vi "SetKparAxisMax.vi"(8 "error in (no error)":errorcluster, 9 "newMax":dbl, 10 "kPar":i32, 11 "dvotAFTKinetics in":refnum<class "dvotAFTKinetics.lvclass">) -> (0 "error out":errorcluster, 3 "dvotAFTKinetics out":refnum<class "dvotAFTKinetics.lvclass">)   [LabVIEW 2012, in "dvotAFTKinetics.lvclass"]
uses:
  dvotAFTKinetics.lvclass
  dvotAFTKinetics.lvclass/dvotAFTKinetics.ctl
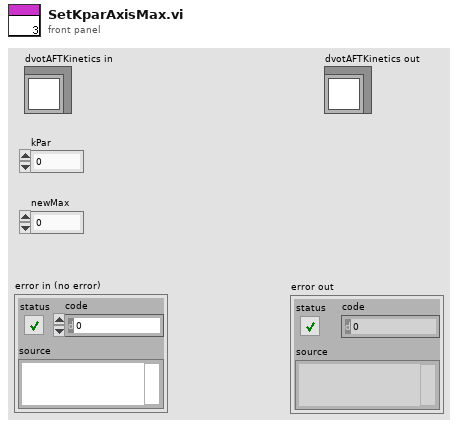
[diagram p1: front panel]
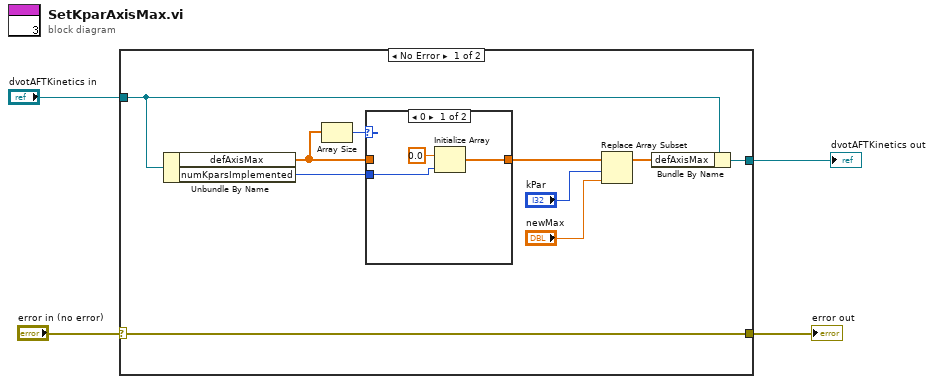
[diagram p0: block diagram]
diagram:
  n1 = case shown="No Error" "error in (no error)" {
    selector: "error in (no error)" -> [w9 w19]
    tunnel: "dvotAFTKinetics in" -> [w14 w20]
    tunnel: [w10 w20] -> w3
    tunnel: [w9 w19] -> w1
    frame No Error {
      n2 = Unbundle By Name(w14) -> ("defAxisMax"=w7:dbl[], "numKparsImplemented"=w5:i32)
      n3 = Array Size(array=w7) -> (size(s)=w8:i32)
      n4 = case shown="0" w8 {
        tunnel: w7 -> [_ w18]
        tunnel: [w17 w18] -> w6
        tunnel: w5 -> [w15 _]
        frame 0 {
          n5 = Initialize Array(0.0 ("element"), w15) -> (w17:dbl[])
        }
        frame Default {
        }
      }
      n6 = Replace Array Subset(array=w6, new element="newMax", index="kPar") -> (w11:dbl[])
      n7 = Bundle By Name(cluster=w14, "defAxisMax"=w11) -> (w10:refnum<class "dvotAFTKinetics.lvclass">)
    }
    frame Error {
    }
  }
  "error out" <- w1
  "dvotAFTKinetics out" <- w3
